vi "1D Fit Projected Function, Gradient, Hessian & Chi2.vi"(0 "parameters":dbl[](array[numeric]), 1 "model function":T4, 2 "NL Fit Method":T2, 5 "Y":dbl[](array[numeric]), 7 "X":dbl[](array[numeric]), 9 "Weights":dbl[](array[numeric]), 11 "Error In":errorcluster, 12 "Parameter Bounds":T3) -> (3 "projected parameters":dbl[](array[numeric]), 4 "best fit":dbl[](array[numeric]), 6 "projected Hessian":T1, 8 "projected gradient":dbl[](array[numeric]), 10 "Chi2":dbl, 14 "number of function calls":i32, 15 "Error Out":errorcluster)   [LabVIEW 2021, in "Fits.lvlib"]
doc: "Grouping VIs used together in the core NL Curve Fitting VI."
uses:
  Fits.lvlib
  <vilib>/gmath/NumericalOptimization/LM model function.ctl
  <vilib>/gmath/NumericalOptimization/LM model function reference.ctl
  Nonlinear Fit Method.ctl
  <vilib>/Analysis/Matrix/Datatypes/RealMatrix.ctl
  <vilib>/gmath/NumericalOptimization/LM_output select.ctl
  <vilib>/gmath/NI_Gmath.lvlib
  <vilib>/Analysis/Matrix/NI_Matrix.lvlib
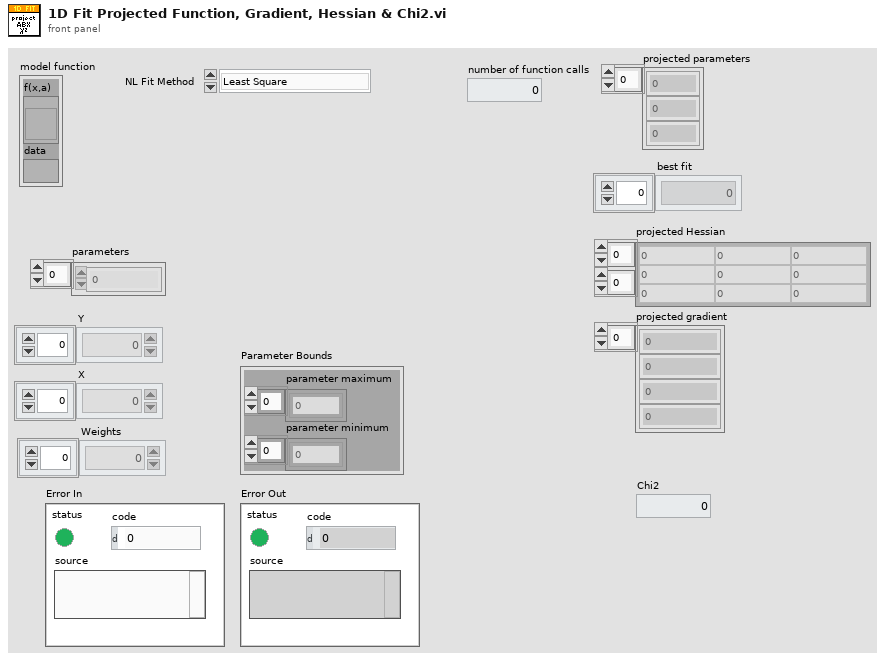
[diagram p1: front panel]
types:
  T1 = typedef "NI_Matrix.lvlib/RealMatrix.ctl" = dbl[][]
  T2 = typedef "Fits.lvlib/Nonlinear Fit Method.ctl" = enum16{"Least Square", "Least Absolute Residual", "Bisquare", "MLE"}
  T3 = cluster{"parameter minimum":dbl[], "parameter maximum":dbl[]}
  T4 = typedef "NI_Gmath.lvlib/LM model function.ctl" = cluster{"f(x,a)":T5, "data":variant}
  T5 = typedef "NI_Gmath.lvlib/LM model function reference.ctl" = refnum<vi>
  T6 = typedef "NI_Gmath.lvlib/LM_output select.ctl" = cluster{"model function":bool, "gradient":bool}
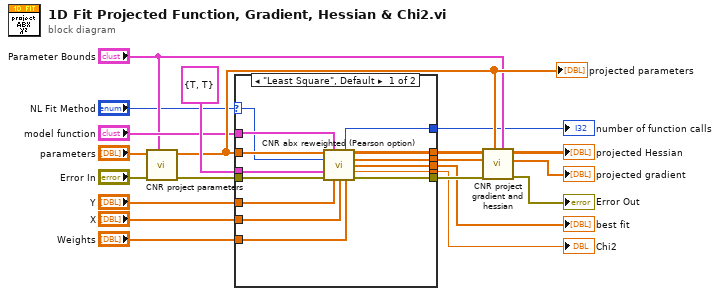
[diagram p0: block diagram]
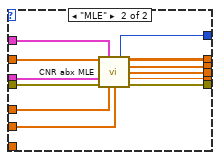
[diagram p2: hidden frame]
diagram:
  n1 = call <vilib>:"CNR project parameters.vi"("bounds"="Parameter Bounds", "error in"="Error In", "parameters"="parameters") -> ("error out"=w19:errorcluster, "projected parameters"=w15:dbl[])  [unwired: 7 out]
  "projected parameters" <- w15
  n2 = case shown="\"Least Square\", Default" "NL Fit Method" {
    selector: "NL Fit Method" -> [w24 _]
    tunnel: "Weights" -> [w34 _]
    tunnel: [w33 w39] -> w2
    tunnel: "model function" -> [w32 w46]
    tunnel: "X" -> [w31 w40]
    tunnel: T6 {"model function"=TRUE, "gradient"=TRUE} ("output control") -> [w30 w44]
    tunnel: w19 -> [w29 w43]
    tunnel: [w28 w42] -> w18
    tunnel: [w27 w36] -> w17
    tunnel: [w26 w37] -> w16
    tunnel: w15 -> [w25 w45]
    tunnel: "Y" -> [w23 w41]
    tunnel: [w22 w38] -> w3
    tunnel: [w21 w35] -> w11
    frame "Least Square", Default {
      n3 = call "CNR abx reweighted (Pearson option).vi"("parameters"=w25, "model function"=w32, "method"=w24, "output control"=w30, "error in (no error)"=w29, "Y"=w23, "X"=w31, "Weight"=w34) -> ("number of function calls"=w21:i32, "Hessian"=w27:T1, "gradient"=w26:dbl[], "best fit"=w22:dbl[], "chiSqr"=w33:dbl, "error out"=w28:errorcluster)  [unwired: 1 in, 1 out]
    }
    frame "MLE" {
      n4 = call "CNR abx MLE.vi"("parameters"=w45, "model function"=w46, "output control"=w44, "error in (no error)"=w43, "Y"=w41, "X"=w40) -> ("number of function calls"=w35:i32, "Hessian"=w36:T1, "gradient"=w37:dbl[], "best fit"=w38:dbl[], "chiSqr"=w39:dbl, "error out"=w42:errorcluster)  [unwired: 3 in, 1 out]
    }
  }
  "number of function calls" <- w11
  "best fit" <- w3
  "Chi2" <- w2
  n5 = call <vilib>:"CNR project gradient and hessian.vi"("bounds"="Parameter Bounds", "projected parameters"=w15, "error in"=w18, "gradient"=w16, "Hessian"=w17) -> ("error out"=→"Error Out":errorcluster, "projected gradient"=→"projected gradient":dbl[], "projected Hessian"=→"projected Hessian":T1)  [unwired: 1 in, 3 out]
